vi "Stop Log.vi"(8 "error in (no error)":errorcluster, 10 "Data":T1, 11 "Log Manager Module in":refnum<class "Log Manager Module.lvclass">) -> (0 "error out":errorcluster, 3 "Log Manager Module out":refnum<class "Log Manager Module.lvclass">)   [LabVIEW 2020, in "VolatusData.lvlib" / "Log Manager Module.lvclass"]
uses:
  Log Manager Module.lvclass
  C:/dev/lv20CE/relink/lv-volatus/Volatus/Module/Module.lvclass
  messages/StopLog/Data.ctl
  Logging State.ctl
  Log Manager Module.lvclass/Log Manager Module.ctl
  Volatus/Module/Module.lvclass/Module.ctl
  Volatus/Event Level.ctl
  Logger State.ctl
  Volatus/MessageQ/MessageQ.lvclass/MessageQ.ctl
  Volatus/Module/Module.lvclass
  VolatusData.lvlib
  Volatus/Volatus.lvlib
  messages/StopLog/StopLog.lvlib
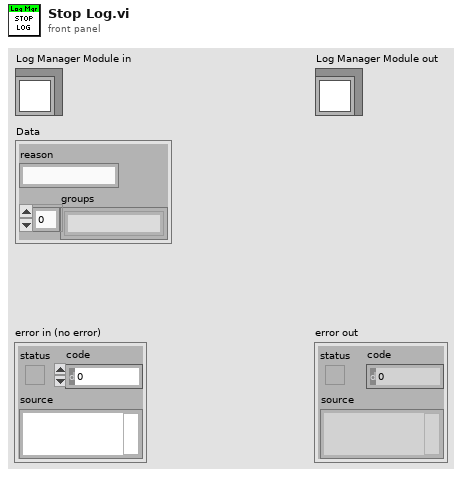
[diagram p1: front panel]
types:
  T1 = typedef "StopLog.lvlib/Data.ctl" = cluster{"reason":string, "groups":string[]}
  T2 = typedef "VolatusData.lvlib/Logging State.ctl" = enum16{"Idle", "Starting", "Logging", "Stopping"}
  T3 = typedef "VolatusData.lvlib/Log Manager Module.lvclass/Group Info.ctl" = cluster{"Name":string, "Loggers":map{string, T4}}
  T4 = typedef "VolatusData.lvlib/Log Manager Module.lvclass/Logger.ctl" = cluster{"ID":string, "MsgQ":refnum<class "MessageQ.lvclass">, "State":T5, "Group":string}
  T5 = typedef "VolatusData.lvlib/Logger State.ctl" = enum16{"Unknown", "Idle", "Preparing", "Ready", "Logging", "Stopping"}
  T6 = typedef "Volatus.lvlib/Event Level.ctl" = enum16{"Debug", "Info", "Warning", "Error"}
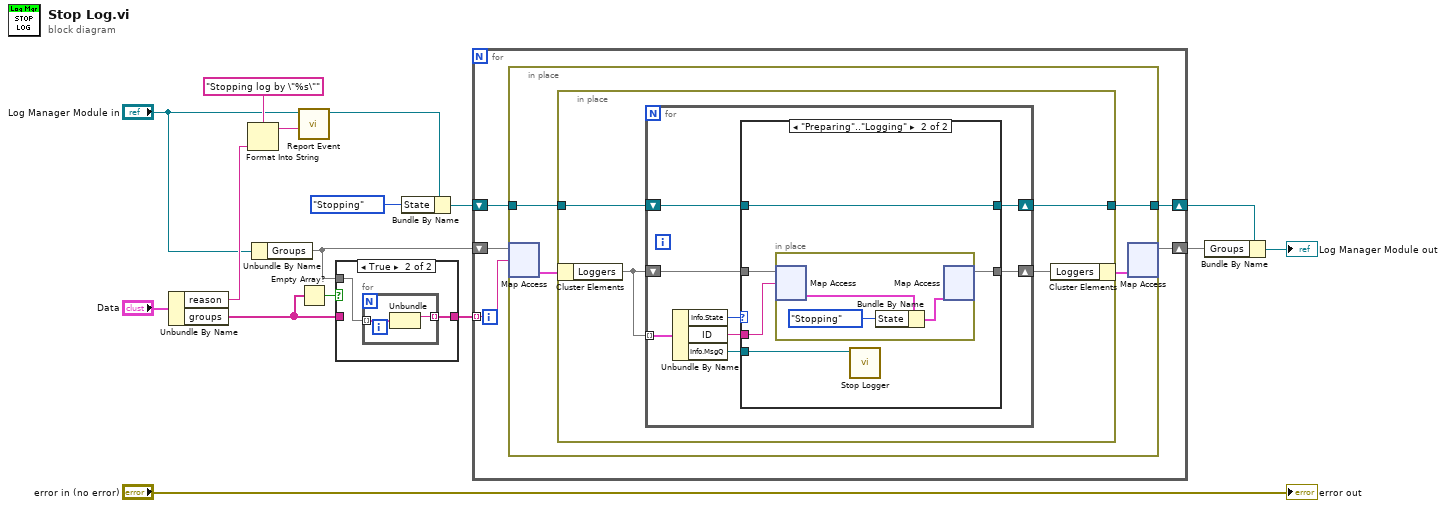
[diagram p0: block diagram]
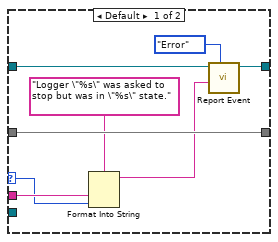
[diagram p2: hidden frame]
diagram:
  n1 = Unbundle By Name("Data") -> ("reason"=w11:string, "groups"=w7:string[])
  n2 = Format Into String(format string="Stopping log by \"%s\"", w11) -> (resulting string=w9:string)  [unwired: 2 in, 1 out]
  n3 = Unbundle By Name("Log Manager Module in") -> ("Groups"=w6:map{string, T3})
  n4 = call "Report Event.vi"("Message"=w9, "Module in"="Log Manager Module in") -> ("Module out"=w1:refnum<class "Log Manager Module.lvclass">)  [unwired: 8 in, 1 out]
  n5 = Empty Array?(array=w7) -> (empty?=w8:bool)
  n6 = case shown="True" w8 {
    tunnel: w7 -> [w17 _]
    tunnel: w6 -> [_ w19]
    tunnel: [w17 w18] -> w5
    frame False {
    }
    frame True {
      n7 = for {
        tunnel: w19 -> [w21] mode=indexing
        tunnel: [w20] -> w18 mode=indexing
        n8 = Unbundle(w21) -> ("Name"=w20:string)  [unwired: 1 out]
      }
    }
  }
  n9 = Bundle By Name(cluster=w1, "State"=Logging_State."Stopping") -> (w3:refnum<class "Log Manager Module.lvclass">)
  n10 = for {
    tunnel: w5 -> [w25] mode=indexing
    shift-right: [w24] -> w14
    shift-left: w6 -> [w26]
    shift-right: [w22] -> w2
    shift-left: w3 -> [w23]
    n11 = in-place {
      in-place-border: w23 -> [w28]
      in-place-border: [w27] -> w22
      n12 = in-place-map #1(w26, w25) -> (w30:T3)  [unwired: 1 in, 1 out]
      n13 = in-place {
        in-place-border: w28 -> [w32]
        in-place-border: [w31] -> w27
        n14 = in-place-cluster #2(w30) -> ("Loggers"=w34:map{string, T4})
        n15 = for {
          tunnel: w34 -> [w42] mode=indexing
          shift-right: [w39] -> w33
          shift-left: w34 -> [w40]
          shift-right: [w35] -> w31
          shift-left: w32 -> [w36]
          n16 = Unbundle By Name(w42) -> ("Info.State"=w37:T5, "ID"=w38:string, "Info.MsgQ"=w41:refnum<class "MessageQ.lvclass">)
          n17 = case shown="\"Preparing\"..\"Logging\"" w37 {
            selector: w37 -> [w44 _]
            tunnel: w41 -> [_ w51]
            tunnel: w40 -> [w50 w55]
            tunnel: [w50 w54] -> w39
            tunnel: w38 -> [w45 w53]
            tunnel: w36 -> [w48 w52]
            tunnel: [w49 w52] -> w35
            frame Default {
              n18 = Format Into String(format string="Logger \"%s\" was asked to stop but was in \"%s\" state.", w45, w44) -> (resulting string=w43:string)  [unwired: 2 in, 1 out]
              n19 = call "Report Event.vi"("Level (Info)"=Event_Level."Error", "Message"=w43, "Module in"=w48) -> ("Module out"=w49:refnum<class "Log Manager Module.lvclass">)  [unwired: 7 in, 1 out]
            }
            frame "Preparing".."Logging" {
              n20 = in-place {
                n21 = in-place-map #3(w55, w53) -> (w58:T4)  [unwired: 1 in, 1 out]
                n22 = Bundle By Name(cluster=w58, "State"=Logger_State."Stopping") -> (w57:T4)
                n23 = in-place-map #3(w57) -> (w54:map{string, T4})  [unwired: 1 in, 2 out]
              }
              n24 = call "Stop Logger.vi"("MsgQ in"=w51) -> ()  [unwired: 9 in, 2 out]
            }
          }
        }
        n25 = in-place-cluster #2("Loggers"=w33) -> (w29:T3)
      }
      n26 = in-place-map #1(w29) -> (w24:map{string, T3})  [unwired: 1 in, 2 out]
    }
  }
  n27 = Bundle By Name(cluster=w2, "Groups"=w14) -> (→"Log Manager Module out":refnum<class "Log Manager Module.lvclass">)
  "error out" <- "error in (no error)"
